vi "Untitled 1.vi"() -> ()   [LabVIEW 2019]
uses:
  <vilib>/Instr/_visa.llb/VISA Configure Serial Port (Instr).vi
panel:
  out "result":u8 format="%x"
  out "Big Array":u8[](array[numeric]) format="%x"
  out "RH":dbl
  out "Temp":dbl
  out "number":u32
  out "subarray":u8[](array[numeric]) format="%x"
  out "value":u8[](array[numeric]) format="%x"
  in  "Array 3":u8[](array[numeric]) format="%04x"
  out "Checksum":u8 format="%x"
  out "return count 2":u32
  out "return count":u32
  in  "Array":u8[](array[numeric]) format="%04x"
  out "data string":string
  # "[0x7E 0x00, 0x7D, 0x31, 0x7D, 0x31, 0x00, 0x00, 0x44, 0x00, 0x00, 0x00, 0x02, 0x00, 0x00, 0x00, 0x06, 0x00, 0x01, 0x86, 0xA0, 0x24, 0x00, 0x46, 0x7E]"
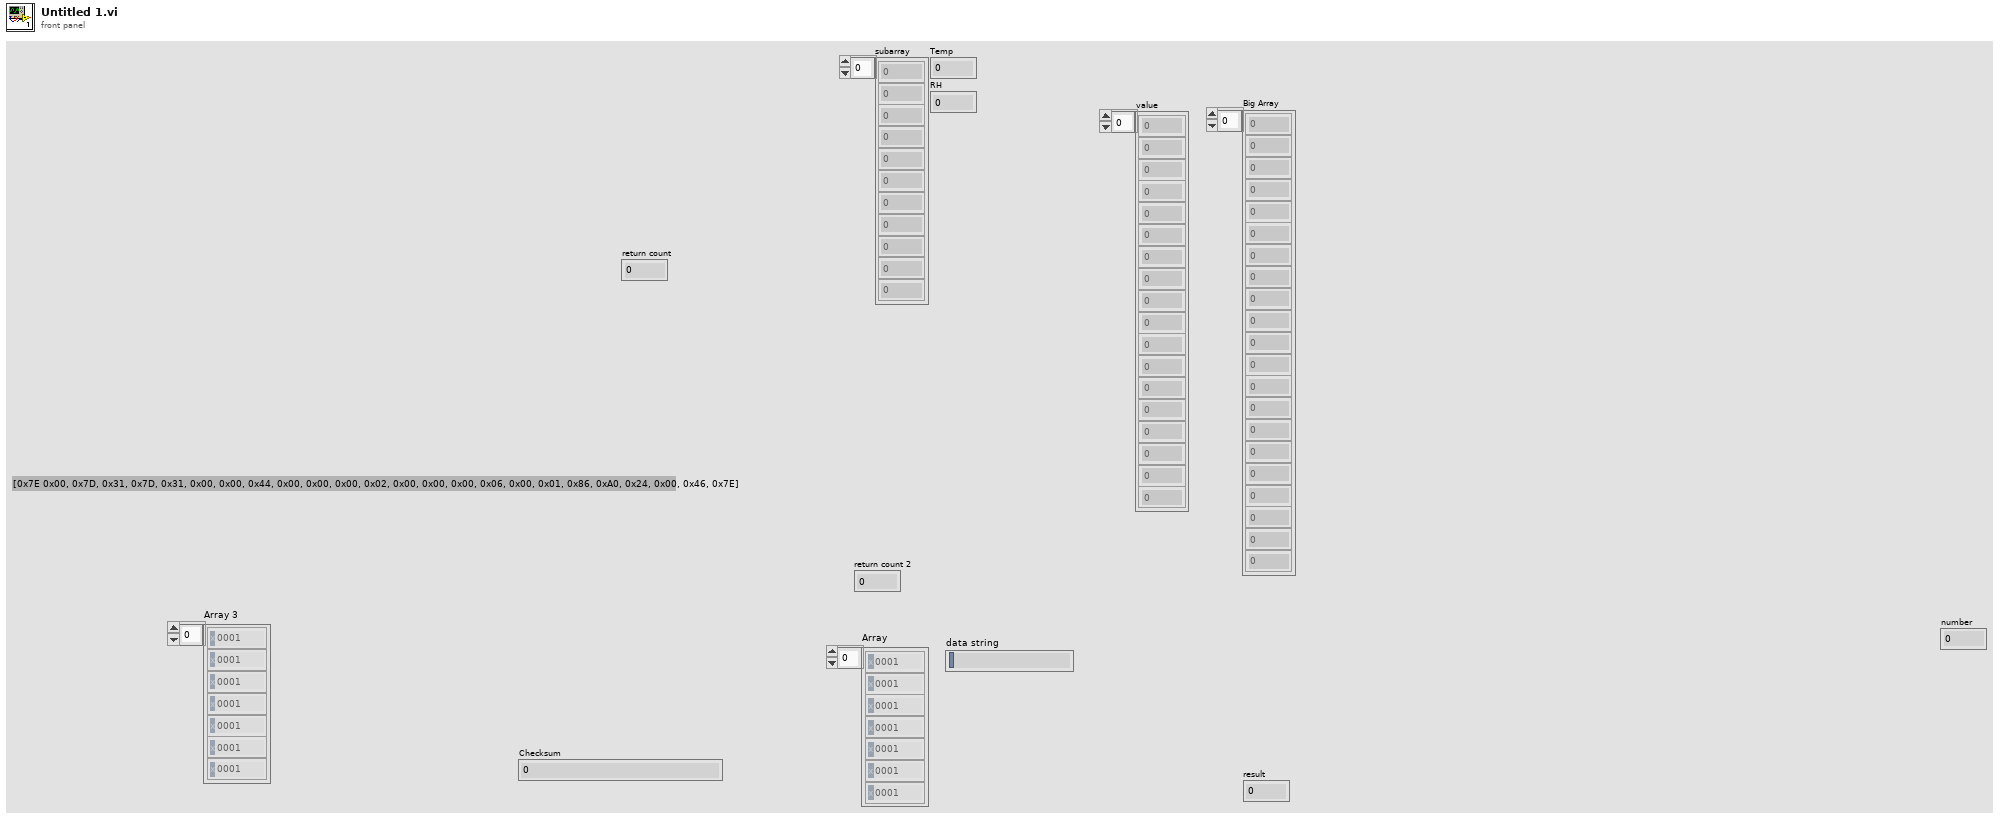
[diagram p1: front panel]
types:
  T1 = enum16{"big-endian, network order", "native, host order", "little-endian"}
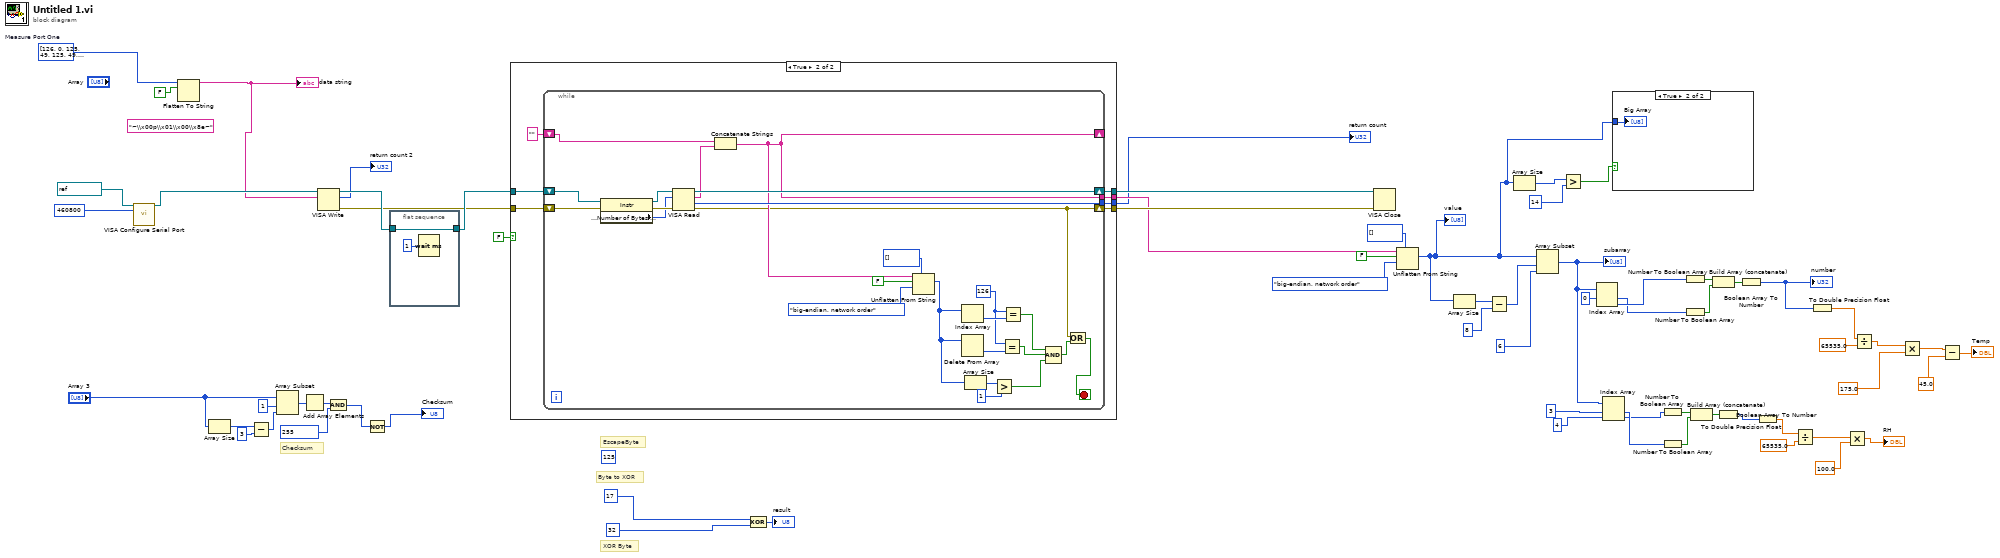
[diagram p0: block diagram]
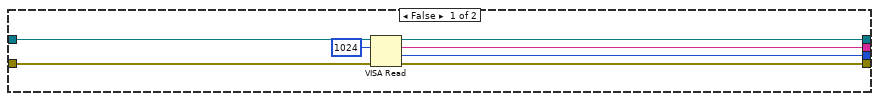
[diagram p2: hidden frame]
diagram:
  (unwired) u8 125
  w42 = u8[] [126, 0, 125, 49, 125, 49, 0, 0, 68, 0, 0, 0, 2, 0, 0, 0, 6, 0, 1, 134, 160, 36, 0, 70, 126]  # Measure Port One
  (unwired) "~\\x00p\\x01\\x00\\x8e~" ("data string 2")
  # "EscapeByte"
  # "Byte to XOR"
  # "XOR Byte"
  # "Checksum"
  n1 = call-poly "VISA Configure Serial Port"("VISA resource name"=refnum<visa-resource-name> "COM7", "baud rate (9600)"=u32 460800) -> ("VISA resource name out"=w56:refnum<visa-resource-name>)  [unwired: 12 in, 1 out]
  n2 = Flatten To String(anything=w42, prepend array or string size? (T)=FALSE) -> (data string=w53:string)  [unwired: 2 in, 2 out]
  "data string" <- w53
  n3 = Array Size(array="Array 3") -> (size(s)=w48:i32)
  n4 = Subtract(x=w48, y=3) -> (x-y=w46:i32)
  n5 = Array Subset(array="Array 3", index=1, length=w46) -> (w49:u8[])
  n6 = Add Array Elements(numeric array=w49) -> (sum=w51:u8)
  n7 = VISA Write(VISA resource name=w56, write buffer=w53) -> (VISA resource name out=w66:refnum<visa-resource-name>, return count=→"return count 2":u32, error out=w62:errorcluster)  [unwired: 1 in]
  n8 = And(x=w51, y=u8 255) -> (x .and. y?=w44:u8)
  n9 = Not(x=w44) -> (.not. x?=→"Checksum":u8)
  n10 = flat-sequence {
    tunnel: w66 -> [w69]
    tunnel: [w69] -> w65
    frame #0 {
      n11 = Wait (ms)(milliseconds to wait=u32 1) -> ()  [unwired: 1 out]
    }
  }
  n12 = case shown="True" FALSE {
    tunnel: w65 -> [w76 w83]
    tunnel: [w75 w82] -> w64
    tunnel: [w73 w81] -> w63
    tunnel: w62 -> [w72 w80]
    tunnel: [w74 w79] -> w61
    tunnel: [w70 w77] -> w9
    frame False {
      n13 = VISA Read(VISA resource name=w76, byte count=u32 1024, error in (no error)=w72) -> (VISA resource name out=w75:refnum<visa-resource-name>, read buffer=w74:string, return count=w70:u32, error out=w73:errorcluster)
    }
    frame True {
      n14 = while {
        tunnel: [w98] -> w79
        tunnel: [w104] -> w77
        shift-right: [w99] -> w82
        shift-left: w83 -> [w107]
        shift-right: [w86] -> w81
        shift-left: w80 -> [w105]
        shift-right: [w98] -> _
        shift-left: "" ("read buffer") -> [w100]
        stop <- w85 stop-if-true
        w95 = u8 126 ("Numeric")
        n15 = property class="Instr"(reference=w107, error in=w105) -> (reference out=w108:refnum<visa-resource-name>, error out=w106:errorcluster, "Serial Settings:Number of Bytes at Serial Port"=w84:u32)
        n16 = VISA Read(VISA resource name=w108, byte count=w84, error in (no error)=w106) -> (VISA resource name out=w99:refnum<visa-resource-name>, read buffer=w88:string, return count=w104:u32, error out=w86:errorcluster)
        n17 = Concatenate Strings(w100, w88) -> (w98:string)
        n18 = Unflatten From String(type=u8[] [] ("Array 2"), binary string=w98, data includes array or string size? (T)=FALSE, byte order (0:big-endian, network order)=T1."big-endian, network order") -> (value=w94:u8[])  [unwired: 1 in, 2 out]
        n19 = Delete From Array(array=w94) -> (deleted portion=w96:u8)  [unwired: 2 in, 1 out]
        n20 = Index Array(array=w94) -> (element=w97:u8)  [unwired: 1 in]
        n21 = Array Size(array=w94) -> (size(s)=w93:i32)
        n22 = Greater?(x=w93, y=1) -> (0:w89:bool)
        n23 = Equal?(x=w95, y=w96) -> (x = y?=w90:bool)
        n24 = Equal?(x=w95, y=w97) -> (x = y?=w91:bool)
        n25 = Compound Arithmetic op=AND(w91, w90, w89) -> (w87:bool)
        n26 = Or(x=w86, y=w87) -> (x .or. y?=w85:bool)
      }
    }
  }
  "return count" <- w9
  n27 = Compound Arithmetic op=XOR(u8 17, u8 32) -> (→"result":u8)
  n28 = VISA Close(VISA resource name=w64, error in (no error)=w63) -> ()  [unwired: 1 out]
  n29 = Unflatten From String(type=u8[] [] ("Array 2"), binary string=w61, data includes array or string size? (T)=FALSE, byte order (0:big-endian, network order)=T1."big-endian, network order") -> (value=w5:u8[])  [unwired: 1 in, 2 out]
  "value" <- w5
  n30 = Array Size(array=w5) -> (size(s)=w41:i32)
  n31 = Subtract(x=w41, y=8) -> (x-y=w39:i32)
  n32 = Array Size(array=w5) -> (size(s)=w8:i32)
  n33 = Array Subset(array=w5, index=w39, length=6) -> (w23:u8[])
  "subarray" <- w23
  n34 = Greater?(x=w8, y=14 ("x")) -> (0:w6:bool)
  n35 = Index Array(array=w23, index #1=0 ("index")) -> (element #1=w24:u8, element #2=w25:u8)  [unwired: 1 in]
  n36 = Index Array(array=w23, index #1=3 ("index"), index #2=4 ("index")) -> (element #1=w17:u8, element #2=w16:u8)
  n37 = case shown="True" w6 {
    tunnel: w5 -> [_ w109]
    frame False {
    }
    frame True {
      "Big Array" <- w109
    }
  }
  n38 = Number To Boolean Array(number=w16) -> (Boolean array=w20:bool[])
  n39 = Number To Boolean Array(number=w17) -> (Boolean array=w21:bool[])
  n40 = Number To Boolean Array(number=w25) -> (Boolean array=w36:bool[])
  n41 = Number To Boolean Array(number=w24) -> (Boolean array=w35:bool[])
  n42 = Build Array (concatenate)(w20, w21) -> (w22:bool[])
  n43 = Build Array (concatenate)(w36, w35) -> (w34:bool[])
  n44 = Boolean Array To Number(Boolean array=w22) -> (number=w15:u32)
  n45 = Boolean Array To Number(Boolean array=w34) -> (number=w33:u32)
  "number" <- w33
  n46 = To Double Precision Float(number=w15) -> (double precision float=w14:dbl)
  n47 = Divide(x=w14, y=65535.0) -> (x/y=w12:dbl)
  n48 = To Double Precision Float(number=w33) -> (double precision float=w31:dbl)
  n49 = Multiply(x=w12, y=100.0) -> (x*y=→"RH":dbl)
  n50 = Divide(x=w31, y=65535.0) -> (x/y=w30:dbl)
  n51 = Multiply(x=w30, y=175.0) -> (x*y=w28:dbl)
  n52 = Subtract(x=w28, y=45.0) -> (x-y=→"Temp":dbl)
